vi "Keithley 648X Series SetupAcquisition.vi"(7 "error in (no error)":errorcluster, 10 "VISA resource name":refnum<visa-resource-name>="Picoammeter") -> (0 "error out":errorcluster, 3 "VISA resource name out":refnum<visa-resource-name>="Picoammeter")   [LabVIEW 2025]
doc: "This example shows how to configure a measurement and take a reading."
uses:
  <instrlib>/Keithley 648X Series/Keithley 648X Series.lvlib
panel:
  in  "Digital Filter Noise Tolerance":dbl
  in  "Enable Digital Filter":u16(ring) items=["Disable", "Enable", "Advanced"]
  in  "Digital Filter Type":u16(ring) items=["Repeating", "Moving"]
  in  "Digital Filter Count":i32=10
  in  "Median Filter Rank":u16(ring)=1 items=["1"=1, "2"=2, "3"=3, "4"=4, "5"=5]
  in  "Enable Median Filter":bool
  in  "Measurement Time":dbl=12.0
  in  "Trigger Delay":dbl
  in  "Trigger Loop Count":i32=1
  in  "Trigger Source":u16(ring) items=["Immediate", "Tlink"]
  in  "Arm Timer Interval":dbl=0.1
  in  "Arm Loop Count":i32=1
  in  "Arm Source":u16(ring) items=["Immediate", "Timer", "Bus", "Tlink", "Manual", "Negative SOT", "Positive SOT", "Bidirectional SOT"]
  # "Note: The product of Arm Loop Count and Trigger Loop Count cannot exceed the maximum non-infinite value that either control can take."
  # "Configure Data Acquisition"
  # "Configure Data Filtration"
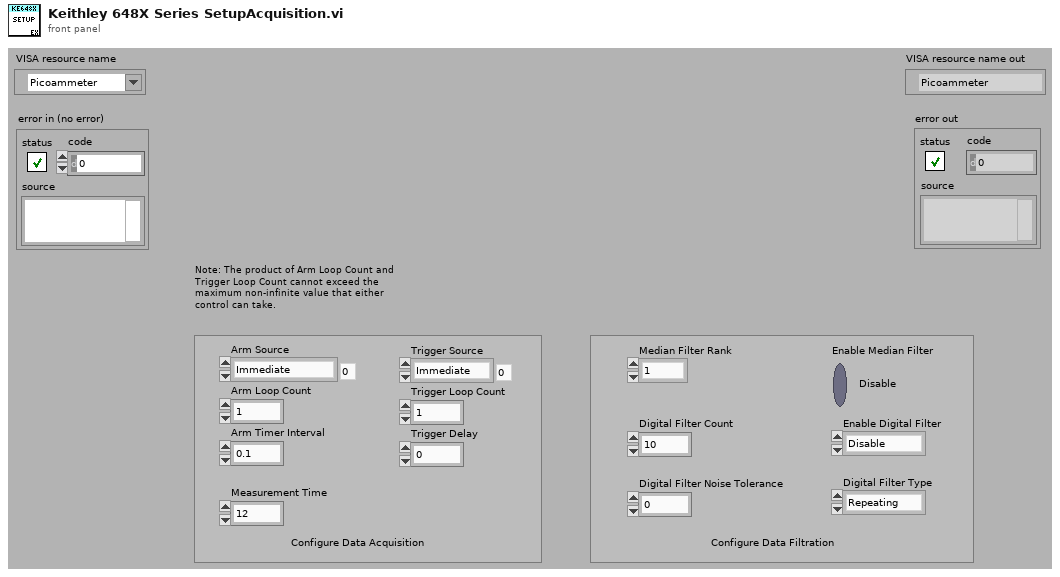
[diagram p1: front panel]
types:
  T1 = cluster{"Baud Rate":u32, "Parity":u16, "Data Bits":u16, "Stop Bits":u16, "Flow Control":u16}
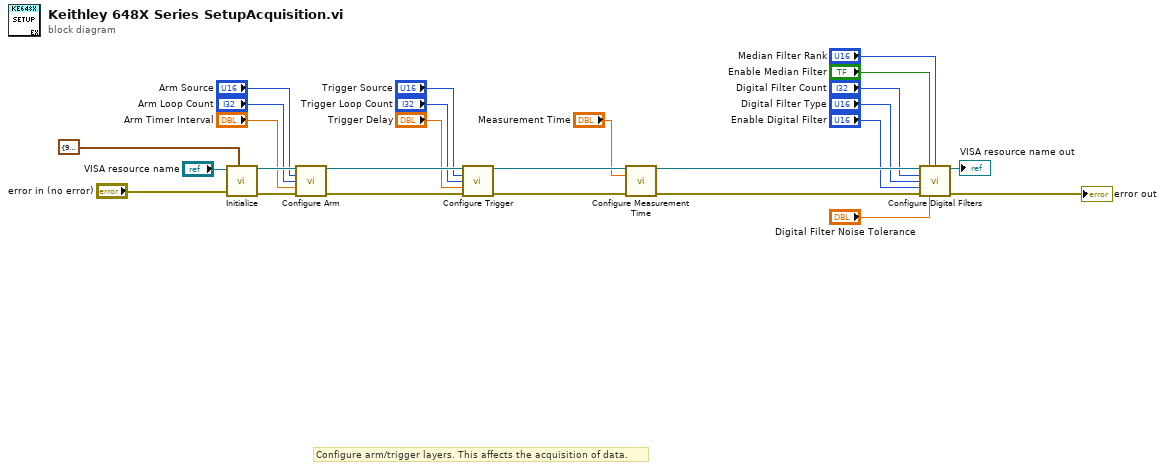
[diagram p0: block diagram]
diagram:
  # "Configure arm/trigger layers. This affects the acquisition of data."
  n1 = call <instrlib>:"Initialize.vi"("Serial Configuration"=T1 {"Baud Rate"=9600, "Parity"=0, "Data Bits"=8, "Stop Bits"=10, "Flow Control"=0}, "error in (no error)"="error in (no error)", "VISA resource name"="VISA resource name") -> ("error out"=w23:errorcluster, "VISA resource name out"=w22:refnum<visa-resource-name>)  [unwired: 7 in]
  n2 = call <instrlib>:"Configure Arm.vi"("VISA resource name"=w22, "Arm Source (0: Immediate)"="Arm Source", "Arm Loop Count (1)"="Arm Loop Count", "Arm Timer Interval (0.1 s)"="Arm Timer Interval", "error in (no error)"=w23) -> ("VISA resource name out"=w21:refnum<visa-resource-name>, "error out"=w24:errorcluster)  [unwired: 9 in]
  n3 = call <instrlib>:"Configure Trigger.vi"("VISA resource name"=w21, "Trigger Source (0: Immediate)"="Trigger Source", "Trigger Loop Count (1)"="Trigger Loop Count", "Trigger Delay (0 s)"="Trigger Delay", "error in (no error)"=w24) -> ("VISA resource name out"=w14:refnum<visa-resource-name>, "error out"=w13:errorcluster)  [unwired: 9 in]
  n4 = call <instrlib>:"Configure Measurement Time.vi"("VISA resource name"=w14, "Measurement Time (6 PLC)"="Measurement Time", "error in (no error)"=w13) -> ("VISA resource name out"=w11:refnum<visa-resource-name>, "error out"=w10:errorcluster)  [unwired: 11 in]
  n5 = call <instrlib>:"Configure Digital Filters.vi"("VISA resource name"=w11, "Enable Median Filter (F: Disable)"="Enable Median Filter", "Median Filter Rank (1)"="Median Filter Rank", "Digital Filter Count (10)"="Digital Filter Count", "Digital Filter Type (0: Repeating)"="Digital Filter Type", "Enable Digital Filter (0: Disable)"="Enable Digital Filter", "error in (no error)"=w10, "Digital Filter Noise Tolerance (0%)"="Digital Filter Noise Tolerance") -> ("VISA resource name out"=→"VISA resource name out":refnum<visa-resource-name>, "error out"=→"error out":errorcluster)  [unwired: 6 in]
